vi "SetLabel.vi"(8 "error in (no error)":errorcluster caption="错误输入（无错误）", 11 "XYPlot 输入":refnum<class "TrendPlot.lvclass">) -> (0 "error out":errorcluster caption="错误输出", 3 "XYPlot 输出":refnum<class "TrendPlot.lvclass">)   [LabVIEW 2018, in "DataDisplay.lvlib" / "TrendPlot.lvclass"]
uses:
  TrendPlot.lvclass
  TrendPlot.lvclass/TrendPlot.ctl
  SubVI/DD_Parameter.vi
  DataDisplay.lvlib
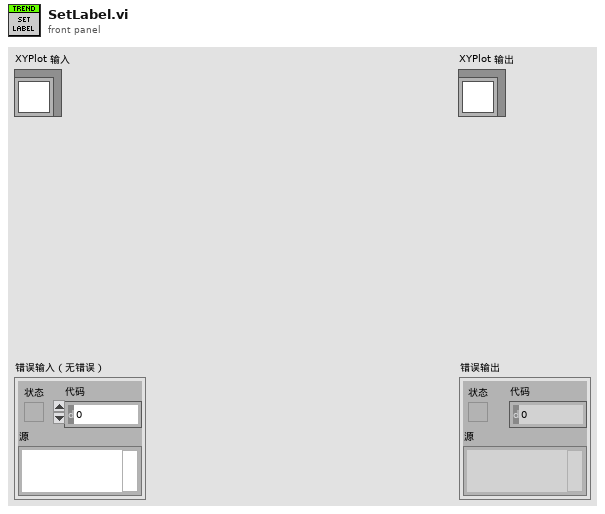
[diagram p1: front panel]
types:
  T1 = typedef "DataDisplay.lvlib/DD_ChannelInfo.ctl" = cluster{"名称":string, "单位":string, "数据类型":enum16{"Real", "Int"}, "趋势线":enum16{"N/A", "X", "Y"}}
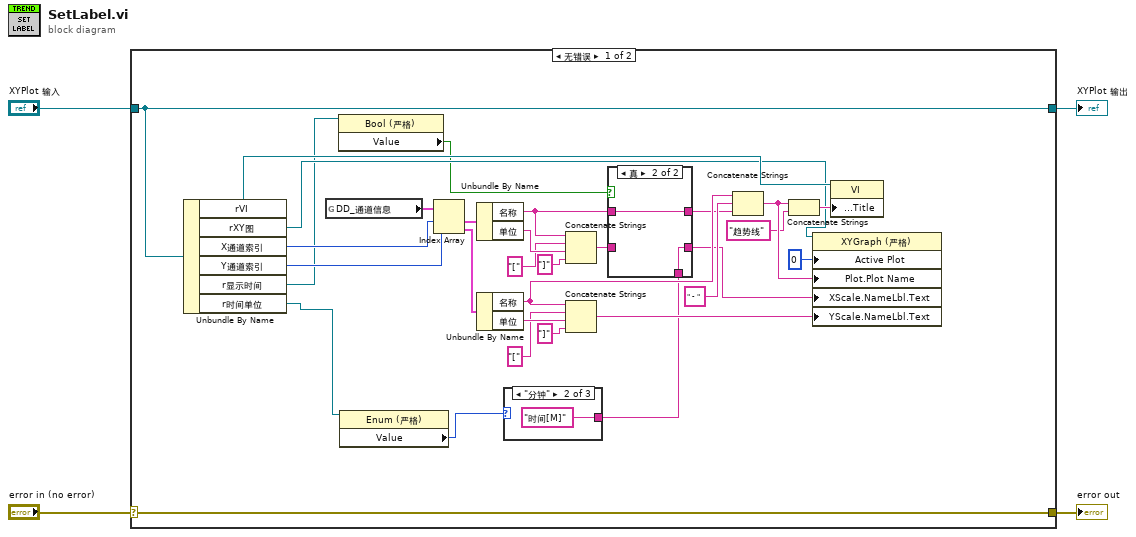
[diagram p0: block diagram]
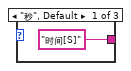
[diagram p2: hidden frame]
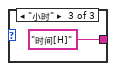
[diagram p3: hidden frame]
diagram:
  n1 = case shown="无错误" "error in (no error)" {
    selector: "error in (no error)" -> [w35 w44]
    tunnel: [w35 w44] -> w3
    tunnel: [w34 w43] -> w1
    tunnel: "XYPlot 输入" -> [w34 w43]
    frame No Error {
      n2 = Unbundle By Name(w34) -> ("rVI"=w19:refnum<vi>, "rXY图"=w18:refnum<vi>, "X通道索引"=w14:i32, "Y通道索引"=w16:i32, "r显示时间"=w9:refnum<vi>, "r时间单位"=w7:refnum<vi>)
      n3 = global read "DD_Parameter.vi" "DD_通道信息"() -> (w17:T1[])
      n4 = property class="Bool (严格)"(reference=w9) -> ("Value"=w8:bool)  [unwired: 1 in, 2 out]
      n5 = property class="Enum (严格)"(reference=w7) -> ("Value"=w6:enum16{"秒", "分钟", "小时"})  [unwired: 1 in, 2 out]
      n6 = Index Array(array=w17, index #1=w14, index #2=w16) -> (element #1=w28:T1, element #2=w29:T1)
      n7 = Unbundle By Name(w28) -> ("名称"=w11:string, "单位"=w30:string)
      n8 = Unbundle By Name(w29) -> ("名称"=w15:string, "单位"=w31:string)
      n9 = case shown="\"分钟\"" w6 {
        tunnel: ["时间[S]" "时间[M]" "时间[H]"] -> w5
        frame "秒", Default {
        }
        frame "分钟" {
        }
        frame "小时" {
        }
      }
      n10 = Concatenate Strings(w11, "[" ("字符串"), w30, "]" ("字符串")) -> (w12:string)
      n11 = Concatenate Strings(w15, "[" ("字符串"), w31, "]" ("字符串")) -> (w32:string)
      n12 = case shown="真" w8 {
        tunnel: w11 -> [w40 w42]
        tunnel: [w40 w42] -> w13
        tunnel: w12 -> [w39 _]
        tunnel: [w39 w41] -> w10
        tunnel: w5 -> [_ w41]
        frame False {
        }
        frame True {
        }
      }
      n13 = Concatenate Strings(w15, " - " ("字符串"), w13) -> (w33:string)
      n14 = Concatenate Strings(w33, "趋势线" ("字符串")) -> (w27:string)
      n15 = property class="XYGraph (严格)"(reference=w18, "Active Plot"=u32 0 ("活动曲线"), "Plot.Plot Name"=w33, "XScale.NameLbl.Text"=w10, "YScale.NameLbl.Text"=w32) -> ()  [unwired: 1 in, 2 out]
      n16 = property class="VI"(reference=w19, "Front Panel.Title"=w27) -> ()  [unwired: 1 in, 2 out]
    }
    frame Error {
    }
  }
  "error out" <- w3
  "XYPlot 输出" <- w1
